vi "Export Definition.vi"(7 "Type":string, 8 "error in (no error)":errorcluster, 9 "Definition Ouptut Path":path, 10 "Name":string, 11 "InsightCM Console Wrapper in":refnum<class "InsightCM Console Wrapper.lvclass">) -> (0 "error out":errorcluster, 3 "InsightCM Console Wrapper out":refnum<class "InsightCM Console Wrapper.lvclass">)   [LabVIEW 2020, in "InsightCM Console Wrapper.lvclass"]
doc: "Exports a specific type definition from the server as a JSON file. You have to enter the the type, name and the output directory for the JSON file.\n\nConsole command -> exportdefinition -t [type] -n [name] -o [output filepath]"
uses:
  InsightCM Console Wrapper.lvclass
  C:/Users/fflores/Documents/GitHub Projects/LabVIEW-CLI-Wrapper/Console Wrapper/Console Wrapper.lvclass
  Console Wrapper/Console Wrapper.lvclass/Console Wrapper.ctl
  Console Wrapper/Write Command Options.vi
  Console Wrapper/Write Command.vi
  Console Wrapper/Console Wrapper.lvclass
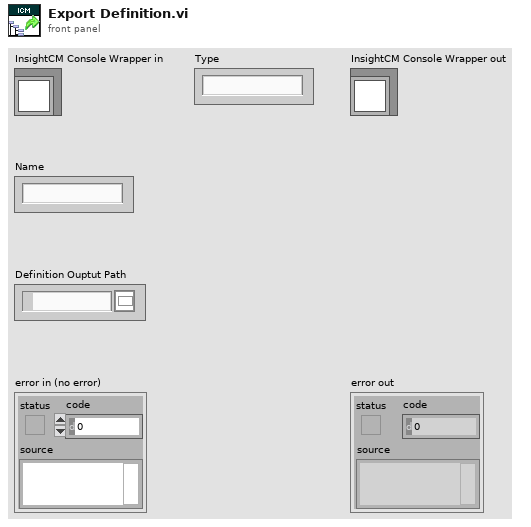
[diagram p1: front panel]
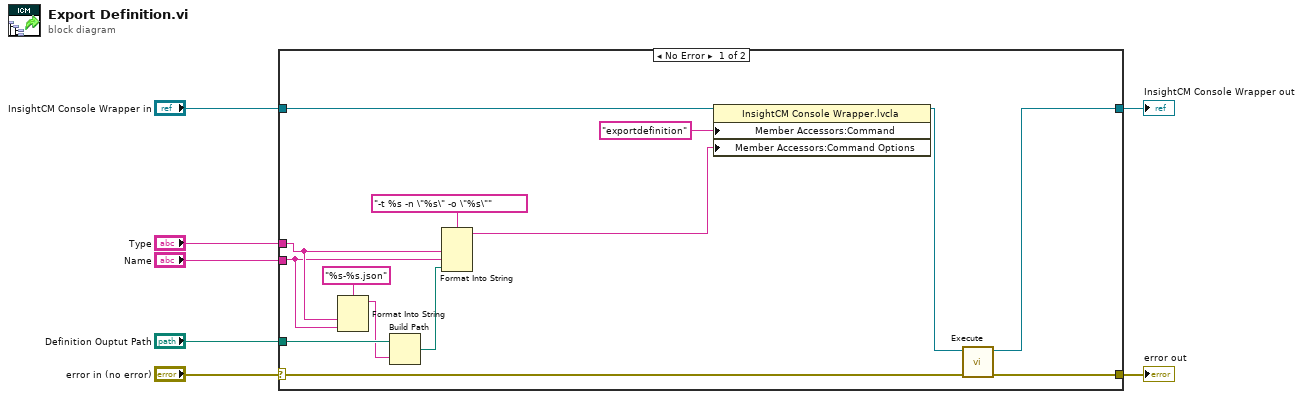
[diagram p0: block diagram]
diagram:
  n1 = case shown="No Error" "error in (no error)" {
    selector: "error in (no error)" -> [w20 w23]
    tunnel: [w18 w23] -> w6
    tunnel: [w16 w22] -> w4
    tunnel: "InsightCM Console Wrapper in" -> [w21 w22]
    tunnel: "Definition Ouptut Path" -> [w10 _]
    tunnel: "Name" -> [w11 _]
    tunnel: "Type" -> [w12 _]
    frame No Error {
      n2 = Format Into String(format string="%s-%s.json", w12, w11) -> (resulting string=w9:string)  [unwired: 2 in, 1 out]
      n3 = Build Path(base path=w10, name or relative path=w9) -> (appended path=w8:path)
      n4 = Format Into String(format string="-t %s -n \"%s\" -o \"%s\"", w12, w11, w8) -> (resulting string=w14:string)  [unwired: 2 in, 1 out]
      n5 = property class="InsightCM Console Wrapper.lvcla"(reference=w21, "Member Accessors:Command"="exportdefinition" ("Command"), "Member Accessors:Command Options"=w14) -> (reference out=w17:refnum<class "InsightCM Console Wrapper.lvclass">)  [unwired: 1 in, 1 out]
      n6 = call "Execute.vi"("error in (no error)"=w20, "Console Wrapper in"=w17) -> ("error out"=w18:errorcluster, "Console Wrapper out"=w16:refnum<class "InsightCM Console Wrapper.lvclass">)  [unwired: 7 in, 1 out]
    }
    frame Error {
    }
  }
  "error out" <- w6
  "InsightCM Console Wrapper out" <- w4
